vi "RM.getDeviceReservationDB.vi"(8 "error in":errorcluster, 11 "Item Ref in":T1 format="%.0x") -> (0 "error out":errorcluster, 1 "found":bool, 2 "reservation DB out":variant, 3 "Item Ref out":T1 format="%.0x")   [LabVIEW 2016, in "FPGA Resource Manager.lvlib"]
uses:
  FPGA Resource Manager.lvlib
  <vilib>/NI Veristand/Custom Device API/Custom Device Item Ref.ctl
  RM.Globals.vi
  <vilib>/NI Veristand/Custom Device API/Get Item Property (Variant).vi
  <vilib>/NI Veristand/Custom Device API/Custom Device API.lvlib
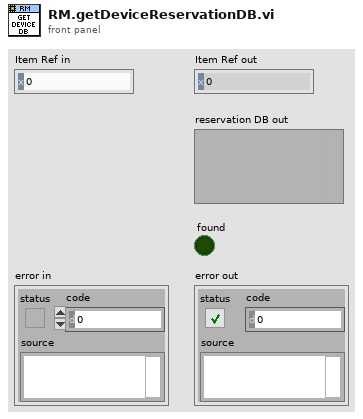
[diagram p1: front panel]
types:
  T1 = typedef "Custom Device API.lvlib/Custom Device Item Ref.ctl" = u64
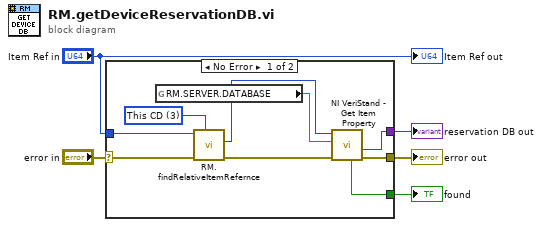
[diagram p0: block diagram]
diagram:
  n1 = case shown="No Error" "error in" {
    selector: "error in" -> [w8 w15]
    tunnel: "Item Ref in" -> [w11 _]
    tunnel: [w13 _] -> w5
    tunnel: [w12 _] -> w4
    tunnel: [w14 w15] -> w3
    frame No Error {
      w9 = u16 3 items=["Targets", "Controller", "Custom Devices", "This CD", "This CD/Group", "This CD/Group/SubGroup"] ("Relative Type")
      n2 = global read "RM.Globals.vi" "RM.SERVER.DATABASE"() -> (w6:string)
      n3 = call "RM.findRelativeItemRefernce.vi"("Relative Type"=w9, "error in (no error)"=w8, "Item Ref in"=w11) -> ("error out"=w7:errorcluster, "Relative Item Ref Out"=w10:T1)  [unwired: 4 in, 3 out]
      n4 = call-poly <vilib>:"NI VeriStand - Get Item Property.vi"("error in (no error)"=w7, "Property Name"=w6, "Item Ref in"=w10) -> ("error out"=w14:errorcluster, "Value"=w13:variant, "Found?"=w12:bool)  [unwired: 5 in, 1 out]
    }
    frame Error {
    }
  }
  "reservation DB out" <- w5
  "found" <- w4
  "error out" <- w3
  "Item Ref out" <- "Item Ref in"
